vi "Print_Control.vi"() -> (1 "Will Print ?":bool, 2 "Return Code":i32)   [LabVIEW 2014]
uses:
  CustomControls/Program_States.ctl
  CustomControls/TSE_Status.ctl
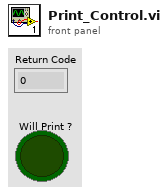
[diagram p1: front panel]
types:
  T1 = typedef "Program_States.ctl" = enum16{"Ön Yükleme", "TSE Baslat", "Kalibratöre Baglan", "Kalibratörü Baslat", "Ön Yükleme Tamam", "Frekans Testi", "Gerilim Testi", "Akim Testi", "Aktif Guc Testi", "Reaktif Guc Testi", "AC Akim Harmonik Testi", "AC Gerilim Harmonik Testi", "Flicker Testi", "Rapor Cikarma", "Yeniden Başlat", "Bekleme", "Durdur"}
  T2 = typedef "TSE_Status.ctl" = cluster{"Return Code":i32, "Message":string, "error in (no error)":errorcluster, "Program State":T1, "Test A. Suresi":u32}
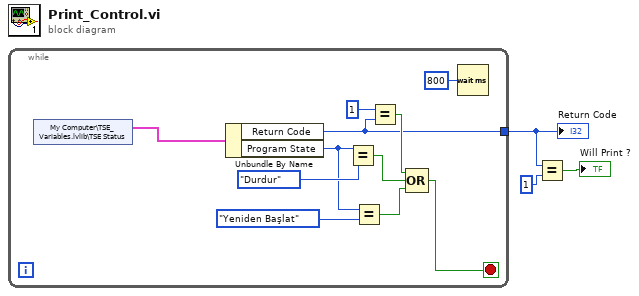
[diagram p0: block diagram]
diagram:
  n1 = while {
    tunnel: [w8] -> w3
    stop <- w13 stop-if-true
    n2 = shared-variable "My Computer\\TSE_Variables.lvlib\\TSE Status"() -> (w11:T2)  [unwired: 1 in, 1 out]
    n3 = Unbundle By Name(w11) -> ("Return Code"=w8:i32, "Program State"=w5:T1)
    n4 = Equal?(x=w5, y=Program_States."Durdur") -> (x = y?=w9:bool)
    n5 = Equal?(x=w5, y=Program_States."Yeniden Başlat") -> (x = y?=w6:bool)
    n6 = Equal?(x=1, y=w8) -> (x = y?=w10:bool)
    n7 = Compound Arithmetic op=OR(w10, w9, w6) -> (w13:bool)
    n8 = Wait (ms)(milliseconds to wait=u32 800) -> ()  [unwired: 1 out]
  }
  "Return Code" <- w3
  n9 = Equal?(x=w3, y=1) -> (x = y?=→"Will Print ?":bool)
